vi "RSZVB Get Receiver Step Attenuators.vi"(8 "error in (no error)":errorcluster {"code" format="%.0x"}, 9 "Analyzer Port (0: Test Port 1)":i32(ring) items=["Test Port 1", "Test Port 2", "Test Port 3", "Test Port 4"], 10 "Channel (1)":i32=1, 11 "VISA session":refnum<visa-resource-name>) -> (0 "error out":errorcluster {"code" format="%.0x"}, 2 "Attenuation Factor":dbl format="%^.3e", 3 "dup VISA session":refnum<visa-resource-name>)   [LabVIEW 2011]
doc: "This VI returns an attenuation factor for the wave received at test port no. <Pt>. The generated wave is attenuated automatically if step attenuators are available.\n\nRemote-control command(s):\n[SENSe<Ch>:]POWer:ATTenuation? ARECeiver | BRECeiver | CRECeiver | DRECeiver"
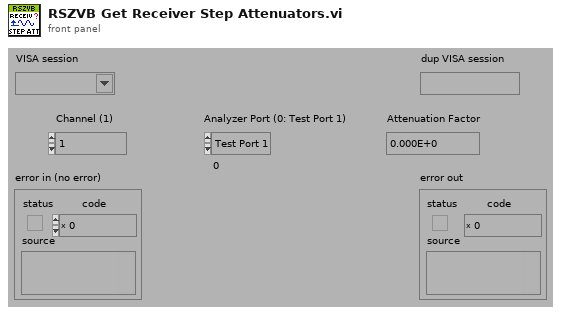
[diagram p1: front panel]
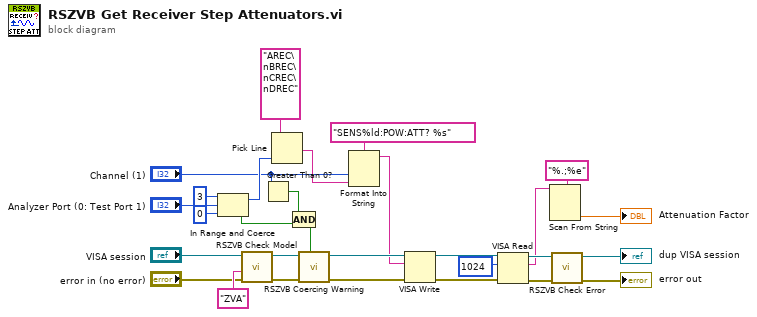
[diagram p0: block diagram]
diagram:
  n1 = In Range and Coerce(upper limit=3, x="Analyzer Port (0: Test Port 1)", lower limit=0) -> (coerced(x)=w19:i32, In Range?=w21:bool)
  n2 = call "RSZVB Check Model.vi"("error in (no error)"="error in (no error)", "Model"="ZVA" ("Options"), "VISA session"="VISA session") -> ("error out"=w4:errorcluster, "dup VISA session"=w3:refnum<visa-resource-name>)  [unwired: 7 in]
  n3 = Greater Than 0?(x="Channel (1)") -> (x > 0?=w24:bool)
  n4 = Pick Line(multi-line string="AREC\nBREC\nCREC\nDREC", line index=w19) -> (output string=w18:string)  [unwired: 1 in]
  n5 = Compound Arithmetic op=AND(w24, w21) -> (w26:bool)
  n6 = call "RSZVB Coercing Warning.vi"("In Range?"=w26, "error in (no error)"=w4, "VISA session"=w3) -> ("error out"=w27:errorcluster, "dup VISA session"=w28:refnum<visa-resource-name>)  [unwired: 7 in]
  n7 = Format Into String(format string="SENS%ld:POW:ATT? %s", "Channel (1)", w18) -> (resulting string=w25:string)  [unwired: 2 in, 1 out]
  n8 = VISA Write(VISA resource name=w28, write buffer=w25, error in (no error)=w27) -> (VISA resource name out=w9:refnum<visa-resource-name>, error out=w10:errorcluster)  [unwired: 1 out]
  n9 = VISA Read(VISA resource name=w9, byte count=u32 1024 ("byte count (0)"), error in (no error)=w10) -> (VISA resource name out=w14:refnum<visa-resource-name>, read buffer=w11:string, error out=w13:errorcluster)  [unwired: 1 out]
  n10 = Scan From String(format string="%.;%e", input string=w11) -> (output 1=→"Attenuation Factor":dbl)  [unwired: 3 in, 3 out]
  n11 = call "RSZVB Check Error.vi"("error in (no error)"=w13, "VISA session"=w14) -> ("error out"=→"error out":errorcluster, "dup VISA session"=→"dup VISA session":refnum<visa-resource-name>)  [unwired: 8 in]
